vi "DestroyTracker.vi"(0 "tracker":u64) -> ()   [LabVIEW 2011]
uses:
  TrackerDLL.vi
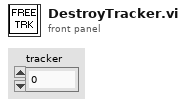
[diagram p1: front panel]
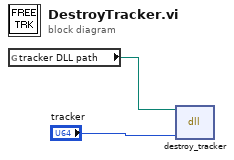
[diagram p0: block diagram]
diagram:
  n1 = global read "TrackerDLL.vi" "tracker DLL path"() -> (w1:path)
  n2 = dll-call lib="D:/jcnossen1/cudaqi-tracker/Debug/cputrack.dll" fn="destroy_tracker"(path in=w1, "tracker"="tracker") -> ()  [unwired: 4 in, 2 out]
